vi "PH_PP_CurrentMeas.contents.vi"   [LabVIEW 2014, in "PH_PP_CurrentMeas.lvlib"]
doc: "This class is forseen to get and indicate the data of the current measurement of the pulsed power at PHELIX. For this purpose it acts on instances of PPMA_DAQClient.\n\nThis class is part of the PHELIX user layer."
uses:
  PH_PP_CurrentMeas.lvlib
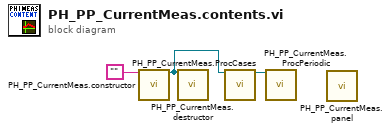
[diagram p0: block diagram]
diagram:
  n1 = call "PH_PP_CurrentMeas.constructor.vi"("name"="") -> ("i ref out"=w1:refnum<vi>)  [unwired: 16 in, 2 out]
  n2 = call "PH_PP_CurrentMeas.destructor.vi"("i ref in"=w1) -> ()  [unwired: 18 in, 1 out]
  n3 = call "PH_PP_CurrentMeas.ProcCases.vi"("i ref in"=w1) -> ("i ref out"=w3:refnum<vi>)  [unwired: 16 in, 2 out]
  n4 = call "PH_PP_CurrentMeas.ProcPeriodic.vi"("i ref in"=w3) -> ()  [unwired: 16 in, 3 out]
  n5 = call "PH_PP_CurrentMeas.panel.vi"() -> ()  [unwired: 19 in, 1 out]
